vi "CLD 6 CSV file utility.vi"(8 "Error In":errorcluster, 10 "[Data In]":T1[](array[typedef])=[{"Dwell Time"=3, "State 1"=TRUE, "State 2"=FALSE, "State 3"=FALSE}, {"Dwell Time"=4, "State 1"=FALSE, "State 2"=TRUE, "State 3"=FALSE}, {"Dwell Time"=5, "State 1"=FALSE, "State 2"=FALSE, "State 3"=TRUE}], 11 "CLD 6 file Enum":T2) -> (0 "Error Out":errorcluster, 3 "[Data Out]":T1[](array[typedef]))   [LabVIEW 2020]
doc: "CLD 6 exercise"
uses:
  Controls/CLD 6 CSV file enum.ctl
  Controls/CLD 6 CSV file data structure.ctl
  <vilib>/Utility/file.llb/Read Delimited Spreadsheet (string).vi
  <vilib>/Utility/file.llb/Write Delimited Spreadsheet (string).vi
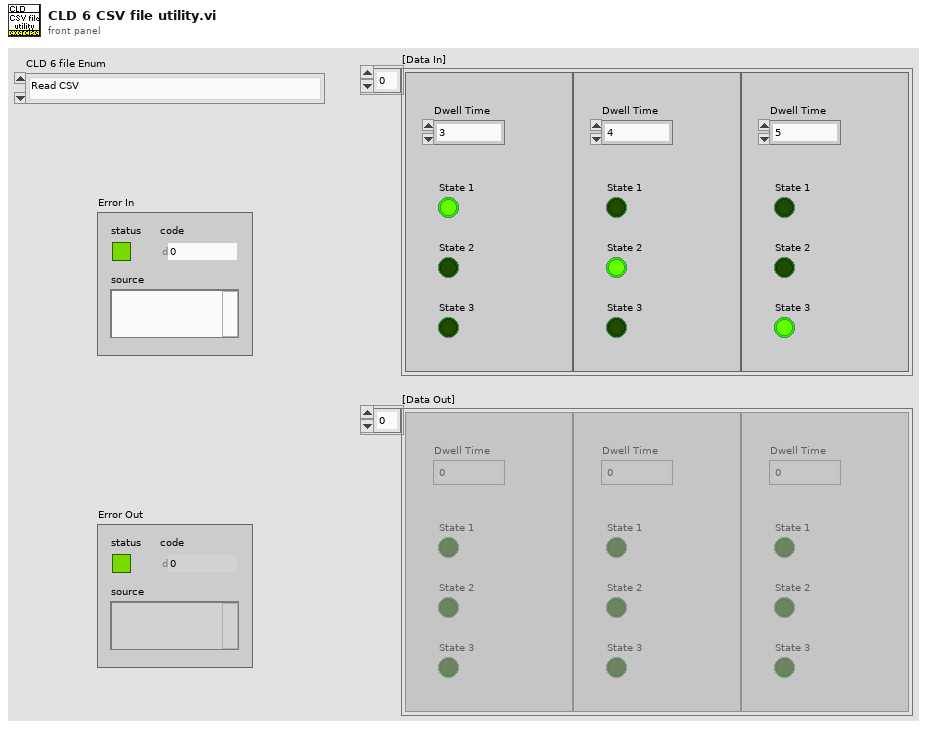
[diagram p1: front panel]
types:
  T1 = typedef "CLD 6 CSV file data structure.ctl" = cluster{"Dwell Time":i32, "State 1":bool, "State 2":bool, "State 3":bool}
  T2 = typedef "CLD 6 CSV file enum.ctl" = enum16{"Read CSV", "Write CSV"}
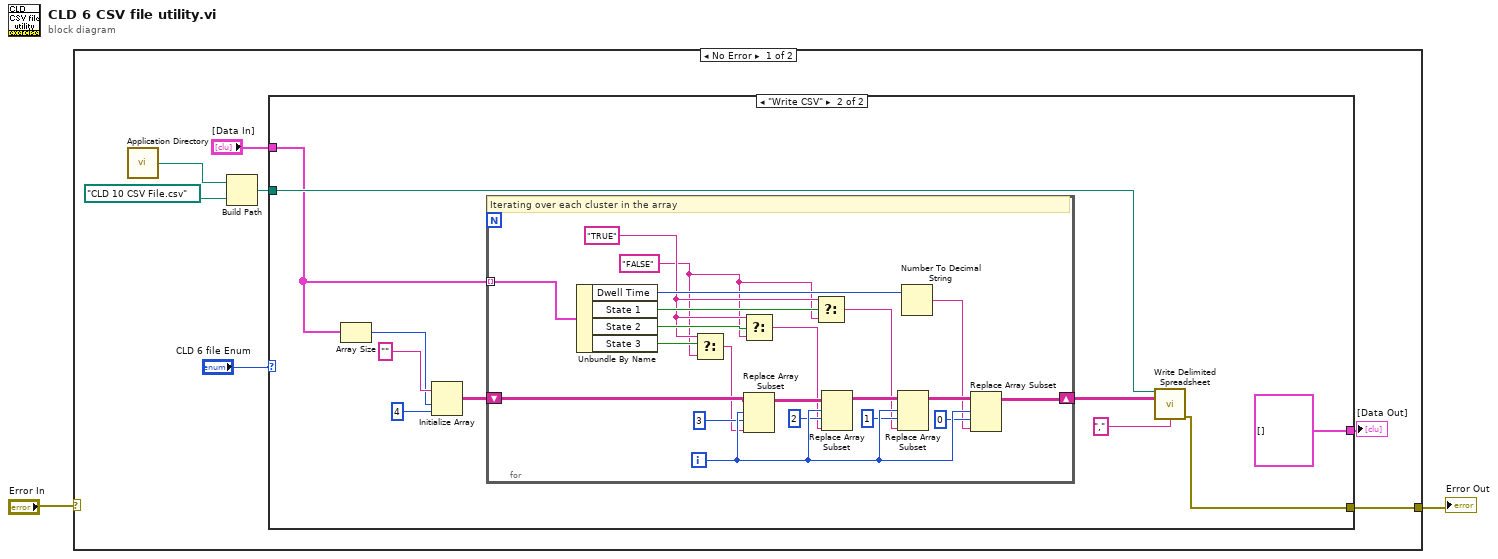
[diagram p0: block diagram]
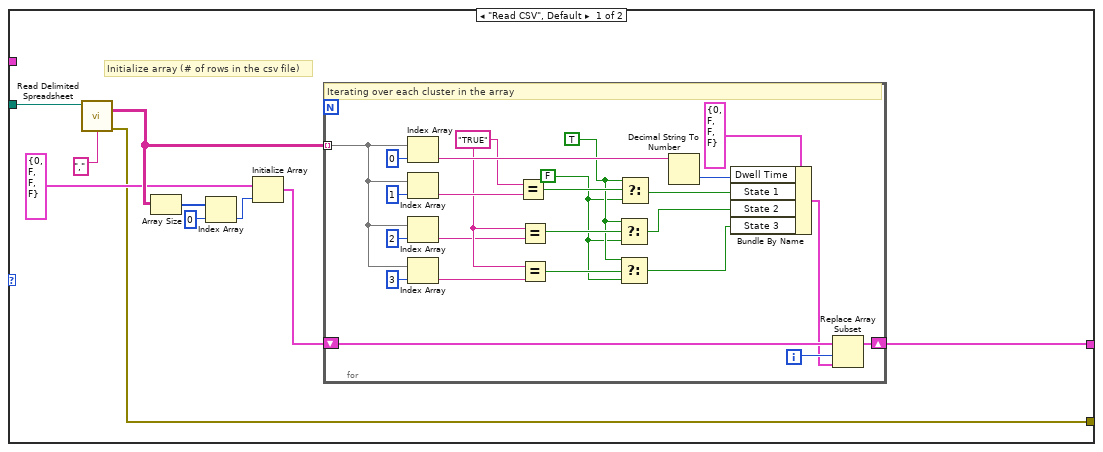
[diagram p2: hidden frame]
diagram:
  n1 = case shown="No Error" "Error In" {
    selector: "Error In" -> [_ w75]
    tunnel: [w3 w75] -> w1
    frame No Error {
      n2 = call <vilib>:"Application Directory.vi"() -> ("Application Directory"=w4:path)
      n3 = Build Path(base path=w4, name or relative path=path "CLD 10 CSV File.csv") -> (appended path=w7:path)
      n4 = case shown="\"Write CSV\"" "CLD 6 file Enum" {
        tunnel: [w10 w48] -> w3
        tunnel: w7 -> [w19 w49]
        tunnel: "[Data In]" -> [_ w44]
        tunnel: [w11 T1[] []] -> w5
        frame "Read CSV", Default {
          # "Initialize array (# of rows in the csv file)"
          n5 = call-poly <vilib>:"Read Delimited Spreadsheet.vi"("file path (dialog if empty)"=w19, "delimiter (\\t)"="," ("delimiter (\\t)")) -> ("all rows"=w17:string[][], "error out"=w10:errorcluster)  [unwired: 8 in, 4 out]
          n6 = Array Size(array=w17) -> (size(s)=w16:i32[])
          n7 = Index Array(array=w16, index=0) -> (element=w14:i32)
          n8 = Initialize Array(T1 {"Dwell Time"=0, "State 1"=FALSE, "State 2"=FALSE, "State 3"=FALSE} ("CSV File Data Structure"), w14) -> (w12:T1[])
          n9 = for {
            tunnel: w17 -> [w42] mode=indexing
            shift-right: [w22] -> w11
            shift-left: w12 -> [w23]
            i -> [w21]
            w27 = FALSE ("f")
            w28 = TRUE
            w34 = "TRUE"
            # "Iterating over each cluster in the array"
            n10 = Index Array(array=w42, index=0) -> (element=w37:string)
            n11 = Index Array(array=w42, index=1) -> (element=w35:string)
            n12 = Index Array(array=w42, index=2) -> (element=w32:string)
            n13 = Index Array(array=w42, index=3) -> (element=w33:string)
            n14 = Equal?(x=w34, y=w35) -> (x = y?=w31:bool)
            n15 = Equal?(x=w34, y=w32) -> (x = y?=w30:bool)
            n16 = Equal?(x=w34, y=w33) -> (x = y?=w29:bool)
            n17 = Select(t=w28, s=w30, f=w27) -> (s? t:f=w25:bool)
            n18 = Select(t=w28, s=w29, f=w27) -> (s? t:f=w24:bool)
            n19 = Select(t=w28, s=w31, f=w27) -> (s? t:f=w26:bool)
            n20 = Decimal String To Number(string=w37) -> (number=w36:i32)  [unwired: 2 in, 1 out]
            n21 = Bundle By Name(cluster=T1 {"Dwell Time"=0, "State 1"=FALSE, "State 2"=FALSE, "State 3"=FALSE} ("CSV File Data Structure"), "Dwell Time"=w36, "State 1"=w26, "State 2"=w25, "State 3"=w24) -> (w20:T1)
            n22 = Replace Array Subset(array=w23, new element=w20, index=w21) -> (w22:T1[])
          }
        }
        frame "Write CSV" {
          n23 = Array Size(array=w44) -> (size(s)=w46:i32)
          n24 = Initialize Array("", w46, 4 ("dimension size")) -> (w51:string[][])
          n25 = for {
            tunnel: w44 -> [w74] mode=indexing
            shift-right: [w68] -> w50
            shift-left: w51 -> [w72]
            i -> [w67]
            w54 = "FALSE"
            w56 = "TRUE"
            # "Iterating over each cluster in the array"
            n26 = Unbundle By Name(w74) -> ("Dwell Time"=w73:i32, "State 1"=w58:bool, "State 2"=w59:bool, "State 3"=w66:bool)
            n27 = Select(t=w56, s=w66, f=w54) -> (s? t:f=w61:string)
            n28 = Select(t=w56, s=w59, f=w54) -> (s? t:f=w57:string)
            n29 = Replace Array Subset(array=w72, new element=w61, index (row)=w67, index (col)=3 ("disabled index (col)")) -> (w71:string[][])
            n30 = Select(t=w56, s=w58, f=w54) -> (s? t:f=w55:string)
            n31 = Replace Array Subset(array=w71, new element=w57, index (row)=w67, index (col)=2 ("disabled index (col)")) -> (w70:string[][])
            n32 = Replace Array Subset(array=w70, new element=w55, index (row)=w67, index (col)=1 ("disabled index (col)")) -> (w69:string[][])
            n33 = Number To Decimal String(number=w73) -> (decimal integer string=w60:string)  [unwired: 1 in]
            n34 = Replace Array Subset(array=w69, new element=w60, index (row)=w67, index (col)=0 ("disabled index (col)")) -> (w68:string[][])
          }
          n35 = call-poly <vilib>:"Write Delimited Spreadsheet.vi"("file path (dialog if empty)"=w49, "2D data"=w50, "delimiter (\\t)"="," ("delimiter (\\t)")) -> ("error out"=w48:errorcluster)  [unwired: 11 in, 1 out]
        }
      }
      "[Data Out]" <- w5
    }
    frame Error {
    }
  }
  "Error Out" <- w1
